vi "Get Size.vi"(11 "Base Graph in":refnum<class "Base Graph.lvclass">) -> (2 "Size":cluster{"Height":u32, "Width":u32}, 3 "Base Graph out":refnum<class "Base Graph.lvclass">)   [LabVIEW 2023, in "Base Graph.lvclass"]
uses:
  Base Graph.lvclass
  Base Graph.lvclass/Base Graph.ctl
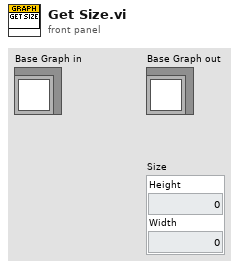
[diagram p1: front panel]
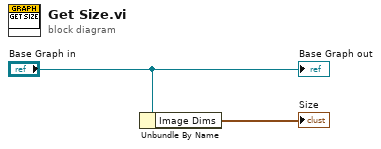
[diagram p0: block diagram]
diagram:
  n1 = Unbundle By Name("Base Graph in") -> ("Image Dims"=→"Size":cluster{"Height":u32, "Width":u32})
  "Base Graph out" <- "Base Graph in"
